vi "Sample_SimpleBoolWrite.vi"() -> ()   [LabVIEW 2022 SP3, in "ADS_Library.lvlib"]
uses:
  ADS_Library.lvlib
panel:
  in  "Boolean":bool
  out "error out":errorcluster
  out "SymbolName":string
  out "bHasMatched":bool
  out "Write Status":bool
  in  "String":string
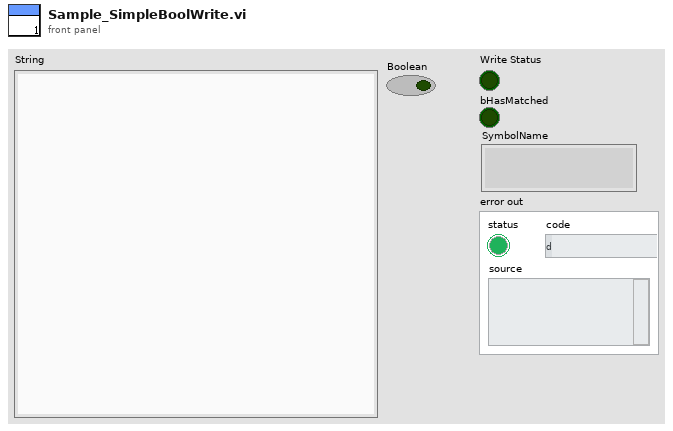
[diagram p1: front panel]
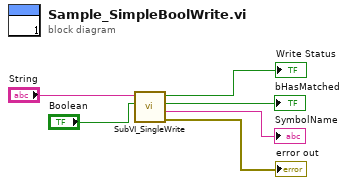
[diagram p0: block diagram]
diagram:
  n1 = call "SubVI_SingleWrite.vi"("WData"="Boolean", "String"="String") -> ("error out"=→"error out":errorcluster, "SymbolName"=→"SymbolName":string, "bHasMatched"=→"bHasMatched":bool, "Write Status"=→"Write Status":bool)  [unwired: 6 in]
